vi "Async Actor.vi"(4 "Queue of Async Elements":refnum<queue>, 9 "Attributes":refnum<class "Attributes.lvclass">, 10 "Unified Actor":refnum<class "Actor.lvclass">) -> ()   [LabVIEW 2025, in "jettl.lvlib"]
uses:
  jettl.lvlib
  Actor/Actor.lvclass
  Attributes/Attributes.lvclass
  Async Elements.ctl
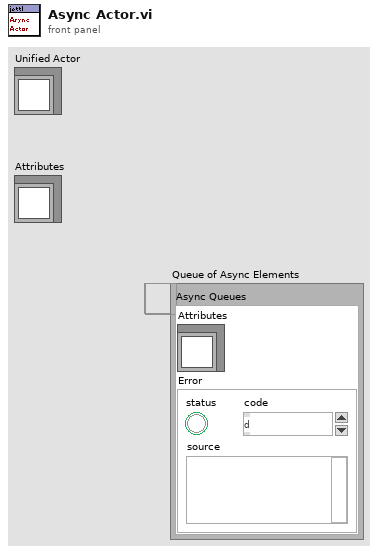
[diagram p1: front panel]
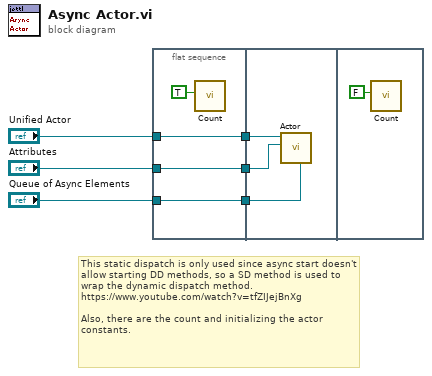
[diagram p0: block diagram]
diagram:
  # "This static dispatch is only used since async start doesn't allow starting DD methods, so a SD method is used to wrap the dynamic dispatch method.\nhttps://www.youtube.com/watch?v=tfZIJejBnXg\n\nAlso, there are the count and initializing the actor constants."
  n1 = flat-sequence {
    tunnel: "Unified Actor" -> [w10]
    tunnel: [w10] -> w5
    tunnel: [w8] -> w4
    tunnel: "Attributes" -> [w8]
    tunnel: [w7] -> w2
    tunnel: "Queue of Async Elements" -> [w7]
    tunnel: w5 -> [w13]
    tunnel: w4 -> [w12]
    tunnel: w2 -> [w11]
    frame #0 {
      n2 = call "Count.vi"("Increment?"=TRUE) -> ()  [unwired: 11 in]
    }
    frame #1 {
      n3 = call-dynamic "Actor.vi"("Queue of Async Elements"=w11, "Attributes"=w12, "Actor in"=w13) -> ()  [unwired: 7 in, 2 out]
    }
    frame #2 {
      n4 = call "Count.vi"("Increment?"=FALSE) -> ()  [unwired: 11 in]
    }
  }
